vi "待机状态数据存储写入和切换量程(子VI).vi"   [LabVIEW 2016, in "斯坦道CODMn.lvlib"]
uses:
  <vilib>/ptbypt/NI_PtbyPt.lvlib
types:
  T1 = cluster{"时间":timestamp, "测量模式":string, "数据类型":string, "检测值":sgl, "单位":string, "数据标识":string, "因子编码":string, "标样参考值":sgl, "ORP-A":sgl, "ORP-B":sgl, "ORP-K":sgl, "COD滴定值":sgl, "高锰酸钾滴定数":sgl, "温度":sgl, "量程":sgl, "LastTime":timestamp, "序列号:":string}
  T2 = cluster{"因子编码":u32, "单位":u16, "标样参考值":sgl, "水样数据时间":timestamp, "水样实测值":sgl, "水样数据标识":string, "标样数据时间":timestamp, "标样实测值":sgl, "标样数据标识":string, "空白数据时间":timestamp, "空白实测值":sgl, "空白数据标识":string, "零点核查数据时间":timestamp, "零点核查实测值":sgl, "零点核查数据标识":string, "跨度核查数据时间":timestamp, "跨度核查实测值":sgl, "跨度核查数据标识":string, "加标回收数据时间":timestamp, "加标回收实测值":sgl, "加标回收数据标识":string, "平行样数据时间":timestamp, "平行样实测值":sgl, "平行样数据标识":string}
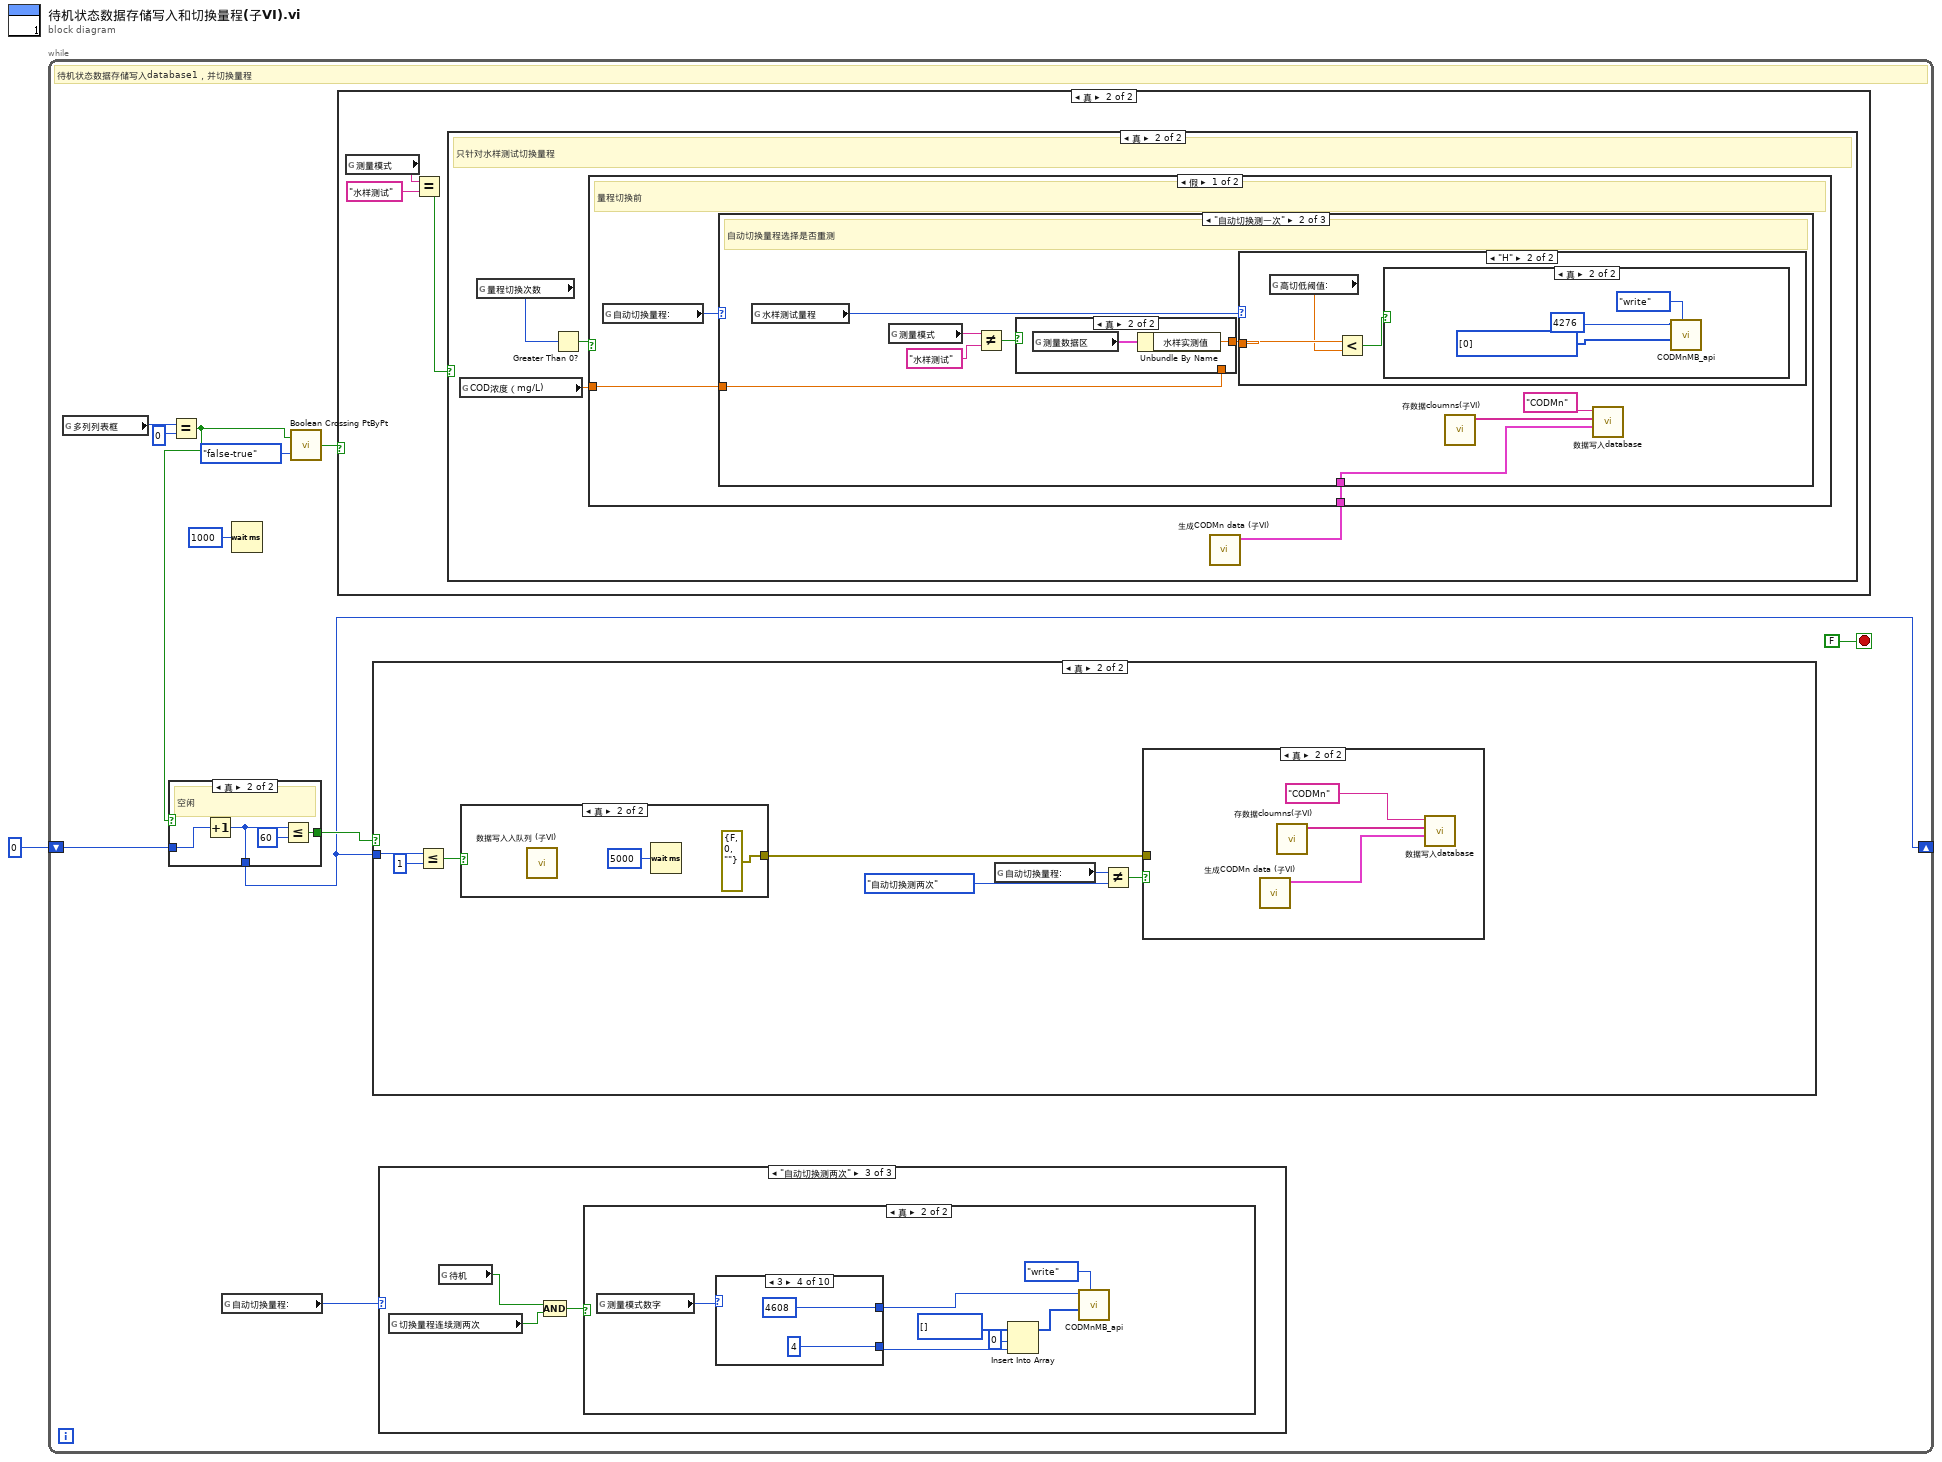
[diagram p0: block diagram]
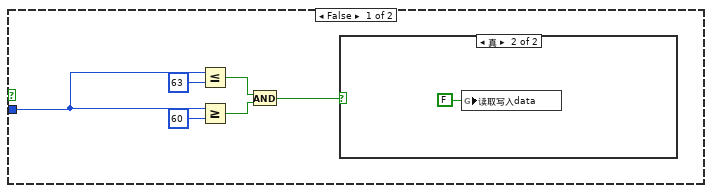
[diagram p2: hidden frame]
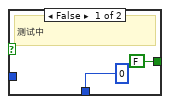
[diagram p6: hidden frame]
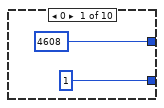
[diagram p10: hidden frame]
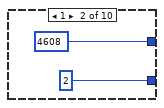
[diagram p11: hidden frame]
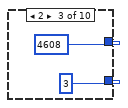
[diagram p12: hidden frame]
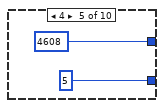
[diagram p13: hidden frame]
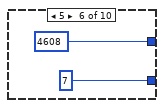
[diagram p14: hidden frame]
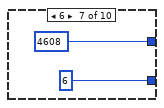
[diagram p15: hidden frame]
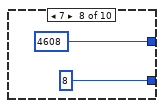
[diagram p16: hidden frame]
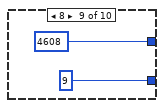
[diagram p17: hidden frame]
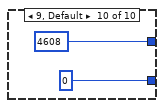
[diagram p18: hidden frame]
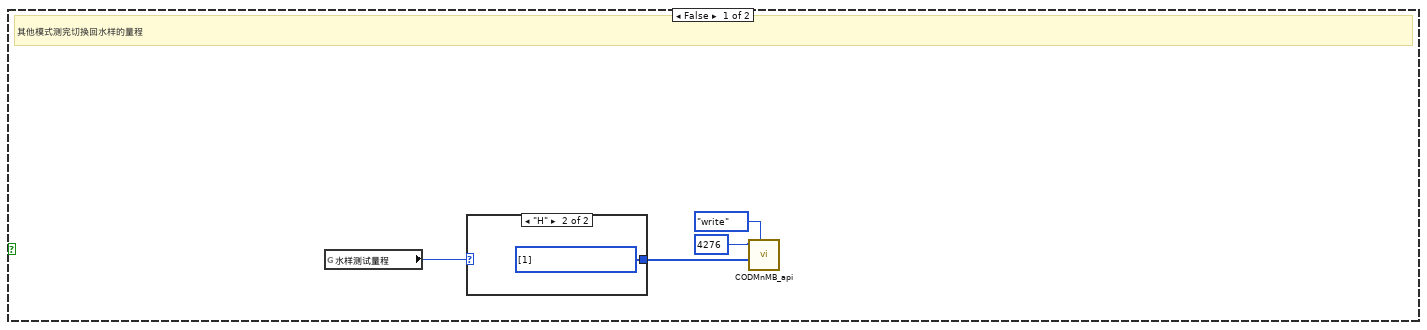
[diagram p20: hidden frame]
diagram:
  n1 = while {
    shift-right: [w2] -> _
    shift-left: 0 ("y") -> [w7]
    stop <- FALSE stop-if-true
    # "待机状态数据存储写入database1，并切换量程"
    n2 = global read "运行时序全局变量.vi" "多列列表框"() -> (w9:i32)
    n3 = Equal?(x=w9, y=0) -> (x = y?=w4:bool)
    n4 = case shown="真" w4 {
      tunnel: w7 -> [_ w36]
      tunnel: [0 w35] -> w2
      tunnel: [FALSE w34] -> w5
      frame False {
        # "测试中"
      }
      frame True {
        # "空闲"
        n5 = Increment(x=w36) -> (x+1=w35:i32)
        n6 = Less Or Equal?(x=w35, y=u32 60) -> (x <= y?=w34:bool)
      }
    }
    n7 = global read "CODMn断电保存全局变量.vi" "自动切换量程:"() -> (w8:enum16{"L", "H", "自动切换测一次", "自动切换测两次"})
    n8 = Wait (ms)(milliseconds to wait=u32 1000 ("等待时间（毫秒）")) -> ()  [unwired: 1 out]
    n9 = call <vilib>:"Boolean Crossing PtByPt.vi"("direction"=enum16{"either", "false-true", "true-false"}."false-true", "input"=w4) -> ("crossing"=w3:bool)  [unwired: 1 in]
    n10 = case shown="真" w3 {
      frame False {
      }
      frame True {
        n11 = global read "COD测量模式全局.vi" "测量模式"() -> (w70:string)
        n12 = Equal?(x=w70, y="水样测试") -> (x = y?=w68:bool)
        n13 = case shown="真" w68 {
          frame False {
            # "其他模式测完切换回水样的量程"
            n14 = global read "CODMn断电保存全局变量.vi" "水样测试量程"() -> (w71:enum16{"L", "H"})
            n15 = case shown="\"H\"" w71 {
              tunnel: [u16[] [0] ("values") u16[] [1] ("values")] -> w72
              frame "L", Default {
              }
              frame "H" {
              }
            }
            n16 = call "CODMnMB_api.vi"("STEP"=enum16{"open", "read", "write", "close"}."write", "values"=w72, "starting address"=u16 4276) -> ()  [unwired: 6 in, 3 out]
          }
          frame True {
            # "只针对水样测试切换量程"
            n17 = global read "COD浓度全局变量.vi" "COD浓度（mg/L)"() -> (w78:dbl)
            n18 = global read "COD内部交互全局.vi" "量程切换次数"() -> (w77:u8)
            n19 = Greater Than 0?(x=w77) -> (x > 0?=w79:bool)
            n20 = call "生成CODMn data (子VI).vi"() -> ("data"=w80:T1)  [unwired: 11 in]
            n21 = case shown="假" w79 {
              tunnel: w80 -> [w83 w141]
              tunnel: w78 -> [w82 _]
              frame False {
                # "量程切换前"
                n22 = global read "CODMn断电保存全局变量.vi" "自动切换量程:"() -> (w81:enum16{"L", "H", "自动切换测一次", "自动切换测两次"})
                n23 = case shown="\"自动切换测一次\"" w81 {
                  tunnel: w83 -> [w84 w89 w115]
                  tunnel: w82 -> [_ w88 w114]
                  frame "H", Default {
                    # "关闭自动切换量程"
                    n24 = call "存数据cloumns(子VI).vi"() -> ("数组"=w86:string[])  [unwired: 11 in]
                    n25 = call "数据写入database.vi"("data"=w84, "columns"=w86, "table"="CODMn") -> ()  [unwired: 8 in, 1 out]
                  }
                  frame "自动切换测一次" {
                    # "自动切换量程选择是否重测"
                    n26 = global read "CODMn断电保存全局变量.vi" "水样测试量程"() -> (w87:enum16{"L", "H"})
                    n27 = global read "COD测量模式全局.vi" "测量模式"() -> (w95:string)
                    n28 = Not Equal?(x=w95, y="水样测试") -> (x != y?=w93:bool)
                    n29 = case shown="真" w93 {
                      tunnel: [w110 w111] -> w92
                      tunnel: w88 -> [w110 _]
                      frame False {
                      }
                      frame True {
                        n30 = global read "CODMn断电保存全局变量.vi" "测量数据区"() -> (w112:T2)
                        n31 = Unbundle By Name(w112) -> ("水样实测值"=w111:sgl)
                      }
                    }
                    n32 = case shown="\"H\"" w87 {
                      tunnel: w92 -> [w99 w105]
                      frame "L", Default {
                        n33 = global read "COD内部交互全局.vi" "高锰酸钾报警"() -> (w96:bool)
                        n34 = global read "CODMn断电保存全局变量.vi" "低切高阈值:"() -> (w97:dbl)
                        n35 = Greater?(x=w99, y=w97) -> (0:w100:bool)
                        n36 = Or(x=w96, y=w100) -> (x .or. y?=w98:bool)
                        n37 = case shown="真" w98 {
                          frame False {
                          }
                          frame True {
                            n38 = call "CODMnMB_api.vi"("STEP"=enum16{"open", "read", "write", "close"}."write", "values"=u16[] [1], "starting address"=u16 4276) -> ()  [unwired: 6 in, 3 out]
                          }
                        }
                      }
                      frame "H" {
                        n39 = global read "CODMn断电保存全局变量.vi" "高切低阈值:"() -> (w104:dbl)
                        n40 = Less?(x=w105, y=w104) -> (x < y?=w106:bool)
                        n41 = case shown="真" w106 {
                          frame False {
                          }
                          frame True {
                            n42 = call "CODMnMB_api.vi"("STEP"=enum16{"open", "read", "write", "close"}."write", "values"=u16[] [0], "starting address"=u16 4276) -> ()  [unwired: 6 in, 3 out]
                          }
                        }
                      }
                    }
                    n43 = call "存数据cloumns(子VI).vi"() -> ("数组"=w91:string[])  [unwired: 11 in]
                    n44 = call "数据写入database.vi"("data"=w89, "columns"=w91, "table"="CODMn") -> ()  [unwired: 8 in, 1 out]
                  }
                  frame "自动切换测两次" {
                    # "自动切换量程选择是否重测"
                    n45 = global read "CODMn断电保存全局变量.vi" "水样测试量程"() -> (w113:enum16{"L", "H"})
                    n46 = case shown="\"H\"" w113 {
                      tunnel: w114 -> [w120 w131]
                      tunnel: w115 -> [w119 w130]
                      frame "L", Default {
                        n47 = global read "CODMn断电保存全局变量.vi" "低切高阈值:"() -> (w117:dbl)
                        n48 = global read "COD内部交互全局.vi" "高锰酸钾报警"() -> (w116:bool)
                        n49 = Greater?(x=w120, y=w117) -> (0:w121:bool)
                        n50 = Or(x=w121, y=w116) -> (x .or. y?=w118:bool)
                        n51 = case shown="真" w118 {
                          tunnel: w119 -> [w122 _]
                          frame False {
                            n52 = call "存数据cloumns(子VI).vi"() -> ("数组"=w124:string[])  [unwired: 11 in]
                            n53 = global write "COD内部交互全局.vi" "data"(w122) -> ()
                            n54 = call "数据写入database.vi"("data"=w122, "columns"=w124, "table"="CODMn") -> ()  [unwired: 8 in, 1 out]
                          }
                          frame True {
                            n55 = global write "COD内部交互全局.vi" "切换量程连续测两次"(TRUE ("切换量程连续测两次")) -> ()
                            n56 = call "CODMnMB_api.vi"("STEP"=enum16{"open", "read", "write", "close"}."write", "values"=u16[] [1], "starting address"=u16 4276) -> ()  [unwired: 6 in, 3 out]
                          }
                        }
                      }
                      frame "H" {
                        n57 = global read "CODMn断电保存全局变量.vi" "高切低阈值:"() -> (w129:dbl)
                        n58 = Less?(x=w131, y=w129) -> (x < y?=w132:bool)
                        n59 = case shown="真" w132 {
                          tunnel: w130 -> [w133 _]
                          frame False {
                            n60 = call "存数据cloumns(子VI).vi"() -> ("数组"=w135:string[])  [unwired: 11 in]
                            n61 = call "数据写入database.vi"("data"=w133, "columns"=w135, "table"="CODMn") -> ()  [unwired: 8 in, 1 out]
                          }
                          frame True {
                            # "重测第一次不存数据"
                            n62 = call "CODMnMB_api.vi"("STEP"=enum16{"open", "read", "write", "close"}."write", "values"=u16[] [0], "starting address"=u16 4276) -> ()  [unwired: 6 in, 3 out]
                            n63 = global write "COD内部交互全局.vi" "切换量程连续测两次"(TRUE ("切换量程连续测两次")) -> ()
                          }
                        }
                      }
                    }
                  }
                }
              }
              frame True {
                # "防止无限切量程"
                n64 = global write "COD内部交互全局.vi" "量程切换次数"(u8 0 ("量程切换次数")) -> ()
                n65 = call "存数据cloumns(子VI).vi"() -> ("数组"=w143:string[])  [unwired: 11 in]
                n66 = call "数据写入database.vi"("data"=w141, "columns"=w143, "table"="CODMn") -> ()  [unwired: 8 in, 1 out]
              }
            }
          }
        }
      }
    }
    n67 = case shown="真" w5 {
      tunnel: w2 -> [w15 w23]
      frame False {
        n68 = Less Or Equal?(x=w15, y=63) -> (x <= y?=w18:bool)
        n69 = Greater Or Equal?(x=w15, y=60) -> (x >= y?=w17:bool)
        n70 = And(x=w18, y=w17) -> (x .and. y?=w13:bool)
        n71 = case shown="真" w13 {
          frame False {
          }
          frame True {
            n72 = global write "COD内部交互全局.vi" "读取写入data"(FALSE ("读取写入data")) -> ()
          }
        }
      }
      frame True {
        n73 = Less Or Equal?(x=w23, y=1) -> (x <= y?=w21:bool)
        n74 = case shown="真" w21 {
          tunnel: [_ errorcluster {"status"=FALSE, "code"=0, "source"=""} ("错误常量")] -> w20
          frame False {
          }
          frame True {
            n75 = call "数据写入入队列 (子VI).vi"() -> ()  [unwired: 12 in]
            n76 = Wait (ms)(milliseconds to wait=u32 5000 ("等待时间（毫秒）")) -> ()  [unwired: 1 out]
          }
        }
        n77 = global read "CODMn断电保存全局变量.vi" "自动切换量程:"() -> (w26:enum16{"L", "H", "自动切换测一次", "自动切换测两次"})
        n78 = Not Equal?(x=w26, y=enum16{"L", "H", "自动切换测一次", "自动切换测两次"}."自动切换测两次") -> (x != y?=w25:bool)
        n79 = case shown="真" w25 {
          tunnel: w20 -> [_ _]
          frame False {
          }
          frame True {
            n80 = call "生成CODMn data (子VI).vi"() -> ("data"=w31:T1)  [unwired: 11 in]
            n81 = call "存数据cloumns(子VI).vi"() -> ("数组"=w30:string[])  [unwired: 11 in]
            n82 = call "数据写入database.vi"("data"=w31, "columns"=w30, "table"="CODMn") -> ()  [unwired: 8 in, 1 out]
          }
        }
      }
    }
    n83 = case shown="\"自动切换测两次\"" w8 {
      frame "H", Default {
      }
      frame "自动切换测一次" {
      }
      frame "自动切换测两次" {
        n84 = global read "COD内部交互全局.vi" "切换量程连续测两次"() -> (w39:bool)
        n85 = global read "COD内部交互全局.vi" "待机"() -> (w38:bool)
        n86 = Compound Arithmetic op=AND ("复合运算")(w38, w39) -> (w40:bool)
        n87 = case shown="真" w40 {
          frame False {
          }
          frame True {
            n88 = global read "COD内部交互全局.vi" "测量模式数字"() -> (w41:i32)
            n89 = case shown="3" w41 {
              tunnel: [u16 4608 ("address") u16 4608 ("address") u16 4608 ("address") u16 4608 ("address") u16 4608 ("address") u16 4608 ("address") u16 4608 ("address") u16 4608 ("address") u16 4608 ("address") u16 4608 ("address")] -> w42
              tunnel: [u16 1 ("address") u16 2 ("address") u16 3 ("address") u16 4 ("address") u16 5 ("address") u16 7 ("address") u16 6 ("address") u16 8 ("address") u16 9 ("address") u16 0 ("address")] -> w47
              frame 0 {
              }
              frame 1 {
              }
              frame 2 {
              }
              frame 3 {
              }
              frame 4 {
              }
              frame 5 {
              }
              frame 6 {
              }
              frame 7 {
              }
              frame 8 {
              }
              frame 9, Default {
              }
            }
            n90 = Insert Into Array(array=u16[] [] ("values"), index=0 ("索引"), new element=w47) -> (w43:u16[])
            n91 = call "CODMnMB_api.vi"("STEP"=enum16{"open", "read", "write", "close"}."write", "values"=w43, "starting address"=w42) -> ()  [unwired: 6 in, 3 out]
          }
        }
      }
    }
  }
